vi "UDcluster to Array.vi"(0 "User-data cluster":T1, 11 "error in (no error)":errorcluster) -> (4 "UD array":string[](array[string]), 15 "error out":errorcluster)   [LabVIEW 2012]
uses:
  typedef/User_Data_Cluster.ctl
  typedef/User Accounts.ctl
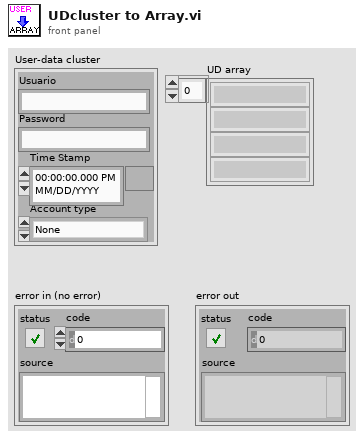
[diagram p1: front panel]
types:
  T1 = typedef "User_Data_Cluster.ctl" = cluster{"Usuario":string, "Password":string, "Account type":T2, "Time Stamp":timestamp}
  T2 = typedef "User Accounts.ctl" = enum16{"None", "User", "Admin"}
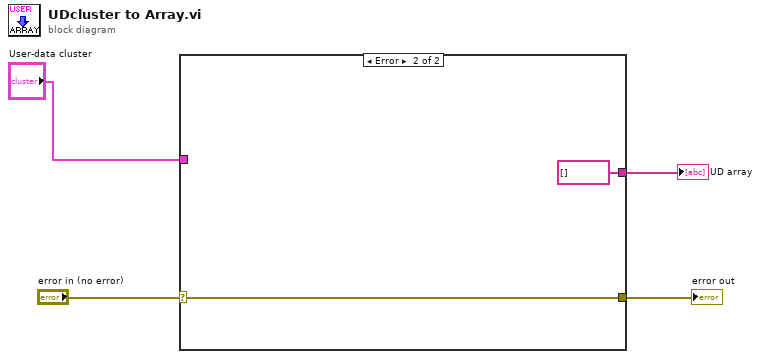
[diagram p0: block diagram]
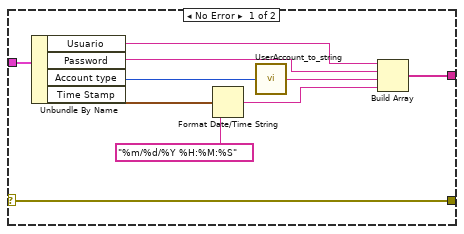
[diagram p2: hidden frame]
diagram:
  n1 = case shown="Error" "error in (no error)" {
    selector: "error in (no error)" -> [w5 w16]
    tunnel: "User-data cluster" -> [w8 _]
    tunnel: [w7 string[] []] -> w4
    tunnel: [w5 w16] -> w2
    frame No Error {
      n2 = Unbundle By Name(w8) -> ("Usuario"=w11:string, "Password"=w6:string, "Account type"=w14:T2, "Time Stamp"=w10:timestamp)
      n3 = Format Date/Time String(time format string (%c)="%m/%d/%Y %H:%M:%S" ("format string"), seconds (now)=w10) -> (date/time string=w13:string)  [unwired: 1 in]
      n4 = call "UserAccount_to_string.vi"("Account"=w14) -> ("String"=w12:string)
      n5 = Build Array(w11, w6, w12, w13) -> (w7:string[])
    }
    frame Error {
    }
  }
  "UD array" <- w4
  "error out" <- w2
